vi "One Identical Inputs.vi"(8 "error in (no error)":errorcluster, 11 "Mock in":refnum<class "Mock.lvclass">) -> (0 "error out":errorcluster, 3 "Mock out":refnum<class "Mock.lvclass">)   [LabVIEW 2020, in "Never.lvclass"]
uses:
  Never.lvclass
  Framework/Mock/Mock.lvclass
  Comparators/Identical Arguments Comparator/Identical Inputs Comparator.lvclass
  C:/git/astemes-lmock/source/Core/Comparator/Comparator.lvclass
  C:/git/astemes-lmock/source/Core/Expectation/Expectation.lvclass
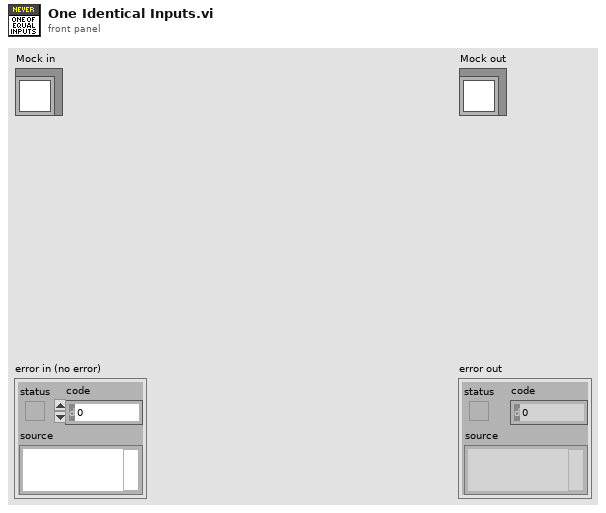
[diagram p1: front panel]
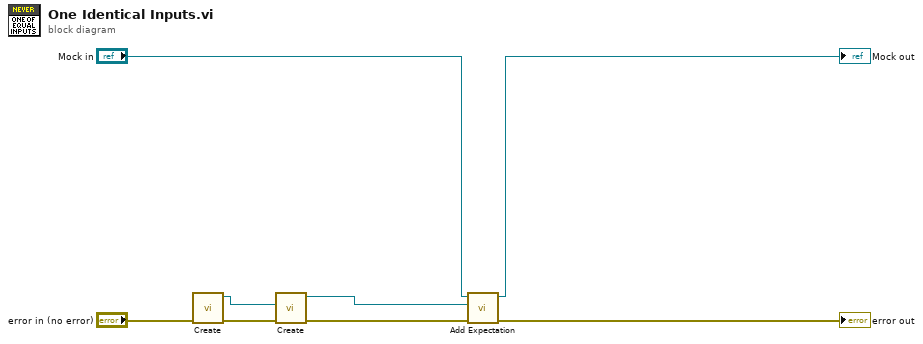
[diagram p0: block diagram]
diagram:
  n1 = call "Create.vi"("error in (no error)"="error in (no error)") -> ("error out"=w1:errorcluster, "Identical Inputs Comparator"=w3:refnum<class "Identical Inputs Comparator.lvclass">)  [unwired: 9 in]
  n2 = call "Create.vi"("error in (no error)"=w1, "Comparator"=w3) -> ("error out"=w5:errorcluster, "One"=w4:refnum<class "Never.lvclass">)  [unwired: 8 in]
  n3 = call-dynamic "Add Expectation.vi"("error in (no error)"=w5, "Expectations"=w4, "Mock in"="Mock in") -> ("error out"=→"error out":errorcluster, "Mock out"=→"Mock out":refnum<class "Mock.lvclass">)  [unwired: 7 in]
